vi "Ignore Warnings.vi"(8 "error in (no error)":errorcluster) -> (0 "error out":errorcluster)   [LabVIEW 2019, in "SEECD Engine.lvlib"]
uses:
  SEECD Engine.lvlib
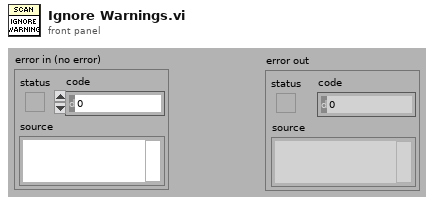
[diagram p1: front panel]
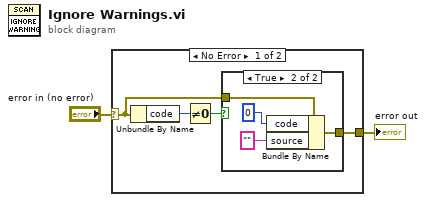
[diagram p0: block diagram]
diagram:
  n1 = case shown="No Error" "error in (no error)" {
    selector: "error in (no error)" -> [w5 w12]
    tunnel: [w6 w12] -> w1
    frame No Error {
      n2 = Unbundle By Name(w5) -> ("code"=w4:i32)
      n3 = Not Equal To 0?(x=w4) -> (x != 0?=w3:bool)
      n4 = case shown="True" w3 {
        tunnel: w5 -> [w7 w11]
        tunnel: [w7 w8] -> w6
        frame False {
        }
        frame True {
          n5 = Bundle By Name(cluster=w11, "code"=0, "source"="") -> (w8:errorcluster)
        }
      }
    }
    frame Error {
    }
  }
  "error out" <- w1
